vi "PicoScope2000aExampleRapidBlockBulkOverlapped.vi"() -> ()   [LabVIEW 2010]
uses:
  shared/PicoBuffers.ctl
  <vilib>/Waveform/DWDTOps.llb/DWDT Analog to Digital.vi
  shared/Segment Range.ctl
  shared/Buffer and Transfer Settings.ctl
  shared/Acquisition Settings.ctl
  shared/nSegments.ctl
  PicoScope2000aLib/PicoScope2000aDigitalChannelSettings.ctl
  PicoScope2000aLib/PicoScope2000aAnalogChannelSettings.ctl
panel:
  in  "roundFaster":bool=TRUE
  out "Pico 2000a Units":string
  in  "Write to TDMS":bool
  in  "timeIntervalRequested":dbl format="%#6_6p"
  out "Properties Panel":T1 {"Max Total Capture Time Available (sec)" format="%.3p"; "Sample Frequency" format="%.3p"; "Sample Internal" format="%.3p"; "Max Samples Available" format="%.3p"; "Total Capture Time (sec)" format="%.3p"}
  in  "Trigger Settings":T2={"Trigger Enabled"=FALSE, "Trigger Source"=enum."Channel A", "Trigger Threshold (Volts)"=0.0, "Trigger Direction"=2, "Trigger Delay (samples)"=0, "Auto Trigger Time (ms)"=1000} {"Trigger Direction" items=["Rising"=2, "Falling"=3]}
  in  "Channel A Settings":T3={"Enabled"=TRUE, "Coupling"=1, "Range"=6, "Analogue Offset"=0.0} {"Analogue Offset" format="%#_6p"; "Range" items=["20 mV"=1, "50 mV"=2, "100 mV"=3, "200 mV"=4, "500 mV"=5, "1 V"=6, "2 V"=7, "5 V"=8, "10 V"=9, "20 V"=10]; "Coupling" items=["AC", "DC"]}
  out "Device Info":T4={"Driver Version"="0", "USB Version"="0", "Hardware"="0", "Variant"="0", "Batch and Serial"="0", "Cal Date"="0", "Kernel Version"="0", "Digital HW Version"="0", "Analogue HW Version"="0", "Firmware 1"="0", "Firmware 2"="0", "MSO"=FALSE, "Number of Channels"=0}
  out "overflow":i16[](array[numeric]) format="%06b"
  in  "Port 0 Settings":T5={"Enabled"=FALSE, "Logic Level"=9830} {"Logic Level" items=["1.5V TTL"=9830, "2.5V CMOS"=16383]}
  in  "Stop Display":bool
  out "Capture Complete":bool
  in  "Run":bool
  in  "Display Buffer Index":i32
  in  "Segment Range":T6={"fromSegmentIndex"=0, "toSegmentIndex"=9} {"toSegmentIndex" format="%.4p"; "fromSegmentIndex" format="%.4p"}
  in  "nSegments":T7=10 format="%.4p"
  out "error out":errorcluster
  in  "Data file":path=path "PicoScope2000aExampleRapidBlock Data"
  in  "Buffer and Transfer Settings":T8={"startIndex"=0, "Samples"=1000, "Down Sample Ratio"=1, "Down-Sample Mode"=0} {"Down-Sample Mode" items=["RAW none"=2147483648, "None"=0, "Aggregate"=1, "Decimate"=2, "Average"=4]; "Down Sample Ratio" step=1; "Samples" format="%_6p"}
  in  "Acquisition Settings":T9={"preTriggerSamples"=0, "postTriggerSamples"=1000, "timebase"=0} {"postTriggerSamples" format="%_6p"; "preTriggerSamples" format="%_6p"}
  out "Port 0":digitalwaveform(graph)={"t0"=timestamp(0 s since 1904-01-01), "dt"=4.800000041882413e-08, "Y"={"transitions"=[], "data"=[]}}
  in  "stop":bool
  out "Analog Channels":cluster{i32, sgl, "Data":dbl[]}[](graph)
  in  "Serial Number":string
  in  "Use Serial Number":bool
  in  "error in (no error)":errorcluster
  # "Number of\nSegments to Capture"
  # "Bit 0 = ChA"
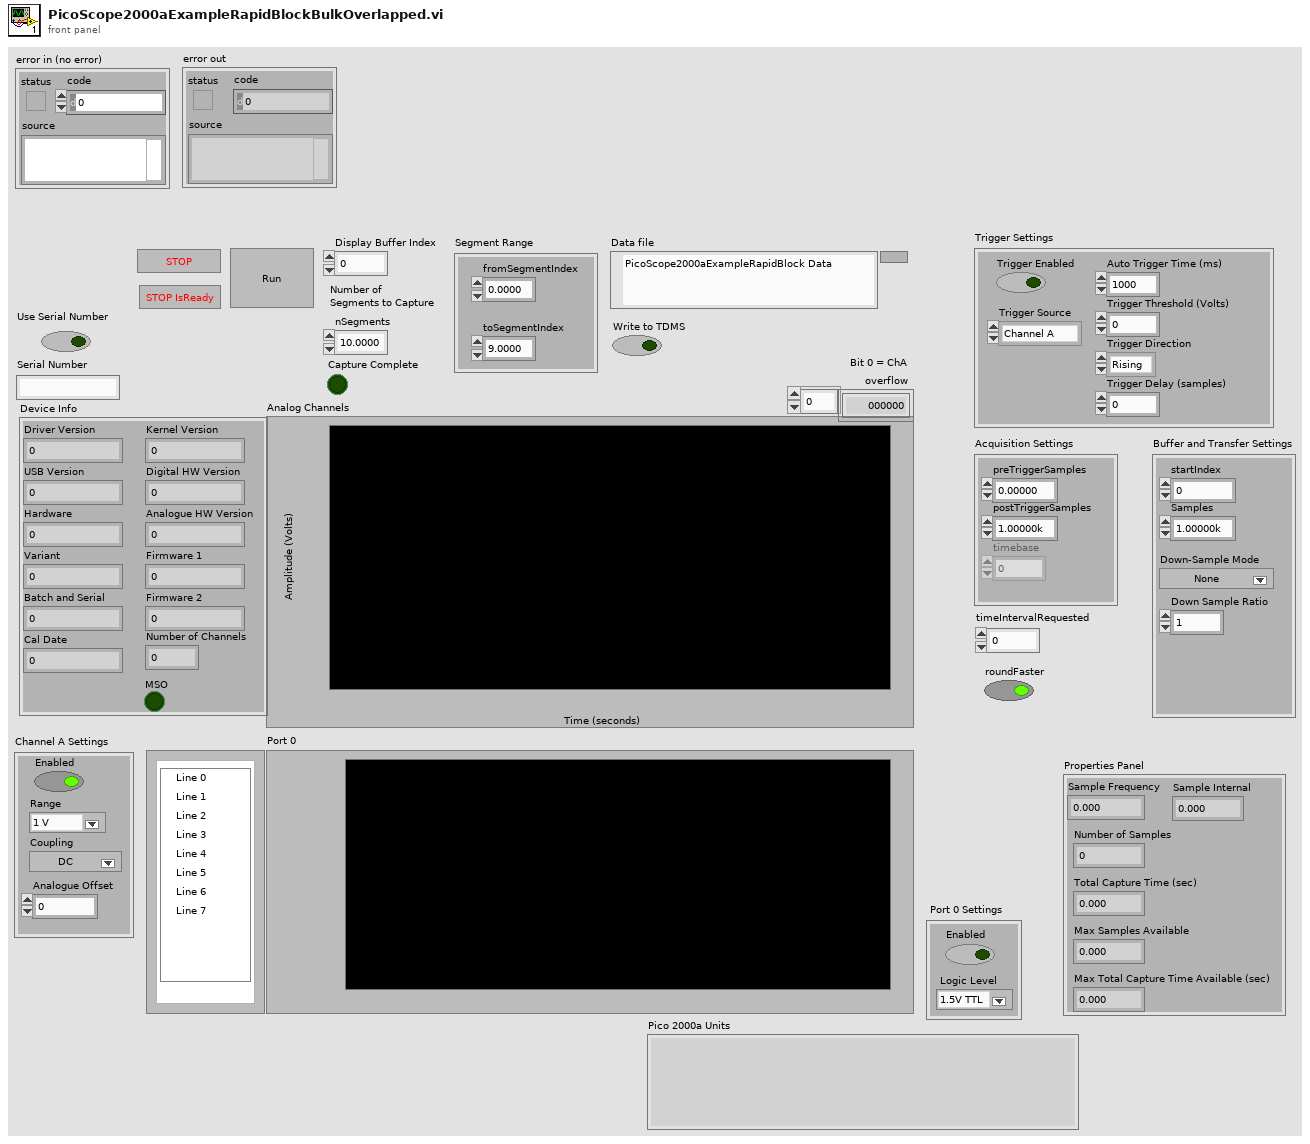
[diagram p1: front panel]
types:
  T1 = cluster{"Sample Frequency":sgl, "Sample Internal":sgl, "Max Samples Available":i32, "Number of Samples":u32, "Total Capture Time (sec) ":sgl, "Max Total Capture Time Available (sec)":sgl}
  T2 = cluster{"Trigger Enabled":bool, "Trigger Source":enum16{"Channel A", "Channel B", "Channel C", "Channel D", "Ext."}, "Trigger Threshold (Volts)":dbl, "Trigger Direction":u16, "Trigger Delay (samples)":u32, "Auto Trigger Time (ms)":i16}
  T3 = typedef "PicoScope2000aAnalogChannelSettings.ctl" = cluster{"Enabled":bool, "Coupling":i16, "Range":u32, "Analogue Offset":sgl}
  T4 = cluster{"Driver Version":string, "USB Version":string, "Hardware":string, "Variant":string, "Batch and Serial":string, "Cal Date":string, "Kernel Version":string, "Digital HW Version":string, "Analogue HW Version":string, "Firmware 1":string, "Firmware 2":string, "MSO":bool, "Number of Channels":i16}
  T5 = typedef "PicoScope2000aDigitalChannelSettings.ctl" = cluster{"Enabled":bool, "Logic Level":i16}
  T6 = typedef "Segment Range.ctl" = cluster{"fromSegmentIndex":u64, "toSegmentIndex":u64}
  T7 = typedef "nSegments.ctl" = u64
  T8 = typedef "Buffer and Transfer Settings.ctl" = cluster{"startIndex":u64, "Samples":u64, "Down Sample Ratio":u64, "Down-Sample Mode":u32}
  T9 = typedef "Acquisition Settings.ctl" = cluster{"preTriggerSamples":u64, "postTriggerSamples":u64, "timebase":u32}
  T10 = typedef "PicoBuffers.ctl" = cluster{"Max Buffer Pointers":u64[][][], "Min Buffer Pointers":u64[][][], "StreamingDataInfo":cluster{"Channel":u32, "Down-Sample Mode":u32, "PICO_DATA_TYPE":enum32{"PICO_INT8_T", "PICO_INT16_T", "PICO_INT32_T", "PICO_UINT32_T", "PICO_INT64_T", ""}, "Samples":i32, "bufferIndex":u64, "startIndex":i32, "overflow":i16}[][]}
  T11 = enum16{"open", "open or create", "create or replace", "create", "open (read-only)"}
  T12 = cluster{"Channel A Buffer":i16[], "Channel B Buffer":i16[], "Channel C Buffer":i16[], "Channel D Buffer":i16[], "Channel E Buffer":i16[], "Channel F Buffer":i16[], "Channel G Buffer":i16[], "Channel H Buffer":i16[], "Port 0 Buffer":i16[], "Port 1 Buffer":i16[]}[]
  T13 = cluster{"Channel A Buffer":i16[], "Channel B Buffer":i16[], "Channel C Buffer":i16[], "Channel D Buffer":i16[], "Channel E Buffer":i16[], "Channel F Buffer":i16[], "Channel G Buffer":i16[], "Channel H Buffer":i16[], "Port 0 Buffer":i16[], "Port 1 Buffer":i16[]}
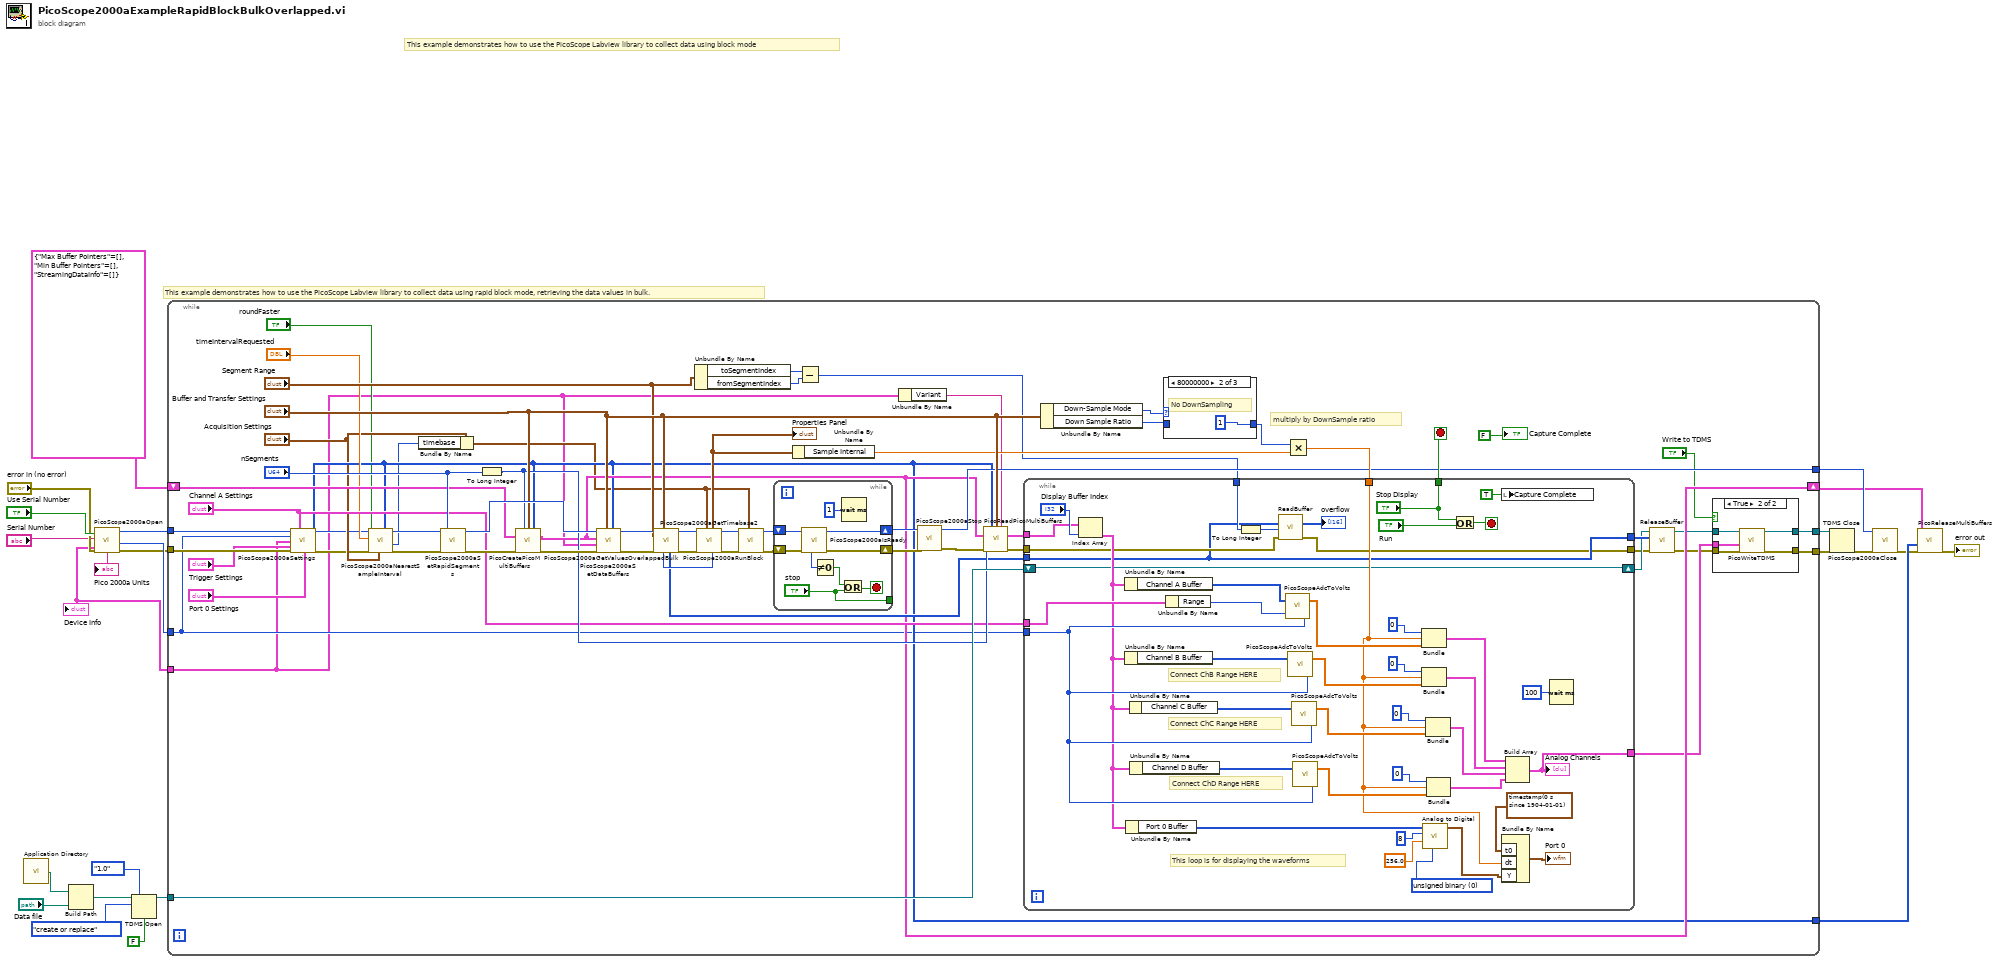
[diagram p0: block diagram]
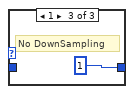
[diagram p4: hidden frame]
diagram:
  # "This example demonstrates how to use the PicoScope Labview library to collect data using rapid block mode, retrieving the data values in bulk."
  # "This example demonstrates how to use the PicoScope Labview library to collect data using block mode"
  n1 = call <vilib>:"Application Directory.vi"() -> ("Application Directory"=w17:path)
  n2 = Build Path(base path=w17, name or relative path="Data file") -> (appended path=w18:path)
  n3 = call "PicoScope2000aOpen.vi"("Serial Number"="Serial Number", "Use Serial Number"="Use Serial Number", "error in (no error)"="error in (no error)") -> ("error out"=w6:errorcluster, "Max Adc value"=w8:i16, "Device Info"=w5:T4, "handle"=w7:i16, "Pico 2000a Units"=→"Pico 2000a Units":string)  [unwired: 3 in, 1 out]
  "Device Info" <- w5
  n4 = TDMS Open(6:FALSE ("disable buffering? (T)"), 7:enum16{"1.0", "2.0"}."1.0" ("file format version (2.0)"), 10:T11."create or replace" ("operation (0:open)"), 11:w18) -> (3:w16:refnum<k34>)  [unwired: 2 in, 1 out]
  n5 = while {
    tunnel: w8 -> [w36]
    tunnel: [w67] -> w23
    tunnel: [w44] -> w24
    tunnel: w16 -> [w86]
    tunnel: [w26] -> w2
    shift-right: [w48] -> w9
    shift-left: T10 {"Max Buffer Pointers"=[], "Min Buffer Pointers"=[], "StreamingDataInfo"=[]} ("Data Pointers") -> [w49]
    tunnel: w7 -> [w38]
    tunnel: w6 -> [w37]
    tunnel: w5 -> [w32]
    tunnel: [w25] -> w3
    stop <- w72 stop-if-true
    # "multiply by DownSample ratio"
    n6 = call "PicoScope2000aSettings.vi"("handle in"=w38, "Channel A Settings"="Channel A Settings", "Max_adc"=w36, "Device Info"=w32, "Trigger Settings"="Trigger Settings", "error in"=w37, "Port 0 Settings"="Port 0 Settings") -> ("handle out"=w39:i16, "Enabled Array"=w44:i16[], "error out"=w40:errorcluster)  [unwired: 6 in]
    n7 = call "PicoScope2000aNearestSampleInterval.vi"("Enabled array"=w44, "Acquisition Settings"="Acquisition Settings", "error in (no error)"=w40, "roundFaster"="roundFaster", "timeIntervalRequested"="timeIntervalRequested", "handle in"=w39) -> ("error out"=w47:errorcluster, "timebase"=w42:u32, "handle out"=w46:i16)  [unwired: 2 in, 1 out]
    n8 = Bundle By Name(cluster="Acquisition Settings", "timebase"=w42) -> (w41:T9)
    n9 = call "PicoScope2000aSetRapidSegments.vi"("nSegments"="nSegments", "error in (no error)"=w47, "handle in"=w46) -> ("error out"=w85:errorcluster, "handle out"=w84:i16)  [unwired: 6 in, 1 out]
    n10 = To Long Integer(number="nSegments") -> (32bit integer=w65:i32)
    n11 = call "PicoCreatePicoMultiBuffers.vi"("Number of Buffers"=w65, "Buffer and Transfer Settings"="Buffer and Transfer Settings", "enabled array"=w44, "Data Pointers In"=w49, "error in (no error)"=w85) -> ("Data Pointers"=w48:T10, "error out"=w87:errorcluster)  [unwired: 9 in]
    n12 = call "PicoScope2000aSetDataBuffers.vi"("enabled array"=w44, "Buffer and Transfer Settings"="Buffer and Transfer Settings", "error in (no error)"=w87, "Device Info"=w32, "Data Pointers In"=w48, "handle in"=w84) -> ("error out"=w83:errorcluster, "handle out"=w82:i16)  [unwired: 4 in]
    n13 = call "PicoScope2000aGetValuesOverlappedBulk.vi"("Segment Range"="Segment Range", "Buffer and Transfer Settings"="Buffer and Transfer Settings", "error in (no error)"=w83, "handle in"=w82) -> ("error out"=w60:errorcluster, "handle out"=w57:i16, "Pointer to Overflow"=w55:u64[], "noOfSamples"=w56:u64)  [unwired: 4 in]
    n14 = Unbundle By Name("Segment Range") -> ("toSegmentIndex"=w53:u64, "fromSegmentIndex"=w52:u64)
    n15 = call "PicoScope2000aGetTimebase2.vi"("Number of Samples"=w56, "Acquisition Settings"=w41, "error in (no error)"=w60, "handle in"=w57) -> ("error out"=w59:errorcluster, "handle out"=w58:i16, "Properties Panel"=w61:T1)  [unwired: 5 in]
    "Properties Panel" <- w61
    n16 = call "PicoScope2000aRunBlock.vi"("Acquisition Settings"=w41, "error in (no error)"=w59, "handle in"=w58) -> ("error out"=w75:errorcluster, "handle out"=w74:i16)  [unwired: 5 in, 2 out]
    n17 = while {
      shift-right: [w145] -> w69
      shift-left: w75 -> [w146]
      shift-right: [w144] -> w66
      shift-left: w74 -> [w143]
      tunnel: ["stop"] -> _
      stop <- w140 stop-if-true
      n18 = call "PicoScope2000aIsReady.vi"("error in (no error)"=w146, "handle in"=w143) -> ("error out"=w145:errorcluster, "handle out"=w144:i16, "ready"=w142:i16)  [unwired: 7 in]
      n19 = Not Equal To 0?(x=w142) -> (x != 0?=w141:bool)
      n20 = Or(x=w141, y="stop") -> (x .or. y?=w140:bool)
      n21 = Wait (ms)(milliseconds to wait=u32 1) -> ()  [unwired: 1 out]
    }
    n22 = Unbundle By Name(w61) -> ("Sample Internal"=w64:sgl)
    n23 = Subtract(x=w53, y=w52) -> (x-y=w50:u64)
    n24 = Unbundle By Name(w32) -> ("Variant"=w63:string)
    n25 = call "PicoScope2000aStop.vi"("error in (no error)"=w69, "handle in"=w66) -> ("error out"=w68:errorcluster, "handle out"=w67:i16)  [unwired: 8 in]
    n26 = call "PicoReadPicoMultiBuffers.vi"("enabled array"=w44, "Buffer and Transfer Settings"="Buffer and Transfer Settings", "Variant"=w63, "Data Pointers"=w48, "No of Buffers"=w65, "error in (no error)"=w68) -> ("MultiBuffers (Max or non-aggregated)"=w80:T12, "error out"=w73:errorcluster)  [unwired: 7 in, 1 out]
    n27 = Unbundle By Name("Buffer and Transfer Settings") -> ("Down-Sample Mode"=w78:u32, "Down Sample Ratio"=w79:u64)
    n28 = case shown="80000000" w78 {
      tunnel: [w147 u64 1 ("Down Sample Ratio") u64 1 ("Down Sample Ratio")] -> w76
      tunnel: w79 -> [w147 _ _]
      frame Default {
      }
      frame -2147483648 {
        # "No DownSampling"
      }
      frame 1 {
        # "No DownSampling"
      }
    }
    n29 = Multiply(x=w76, y=w64) -> (x*y=w77:sgl)
    n30 = while {
      tunnel: w36 -> [w104]
      tunnel: "Channel A Settings" -> [w137]
      tunnel: w80 -> [w114]
      tunnel: w77 -> [w106]
      shift-right: [w95] -> w29
      shift-left: w86 -> [w95]
      tunnel: w73 -> [w100]
      tunnel: ["Stop Display"] -> w72
      tunnel: w55 -> [w98]
      tunnel: [w98] -> w54
      tunnel: w50 -> [w99]
      tunnel: [w97] -> w31
      tunnel: [w96] -> w28
      stop <- w117 stop-if-true
      w128 = u16 0 items=["unsigned binary", "offset binary", "2's complement"] ("data format (offset binary)")
      # "This loop is for displaying the waveforms"
      # "Connect ChB Range HERE"
      # "Connect ChD Range HERE"
      # "Connect ChC Range HERE"
      n31 = Index Array(array=w114, index="Display Buffer Index") -> (element=w103:T13)
      n32 = Unbundle By Name(w103) -> ("Channel A Buffer"=w121:i16[])
      n33 = Unbundle By Name(w103) -> ("Channel B Buffer"=w133:i16[])
      n34 = Unbundle By Name(w103) -> ("Port 0 Buffer"=w126:i16[])
      n35 = Unbundle By Name(w103) -> ("Channel C Buffer"=w112:i16[])
      n36 = Unbundle By Name(w103) -> ("Channel D Buffer"=w108:i16[])
      n37 = Unbundle By Name(w137) -> ("Range"=w135:u32)
      n38 = To Long Integer(number=w99) -> (32bit integer=w102:i32)
      n39 = call "ReadBuffer.vi"("Pointer and BufferSize"=w98, "Buffer size"=w102, "error in (no error)"=w100) -> ("Output Array"=→"overflow":i16[], "error out"=w96:errorcluster)  [unwired: 11 in]
      n40 = call "PicoScopeAdcToVolts.vi"("Max_adc"=w104, "Range Index"=w135, "Data"=w121) -> ("Data"=w122:dbl[])
      n41 = call "PicoScopeAdcToVolts.vi"("Max_adc"=w104, "Data"=w133) -> ("Data"=w132:dbl[])  [unwired: 1 in]
      n42 = call "PicoScopeAdcToVolts.vi"("Max_adc"=w104, "Data"=w112) -> ("Data"=w111:dbl[])  [unwired: 1 in]
      n43 = call "PicoScopeAdcToVolts.vi"("Max_adc"=w104, "Data"=w108) -> ("Data"=w107:dbl[])  [unwired: 1 in]
      n44 = Bundle(0, w106, "Data"=w122) -> (w131:cluster{i32, sgl, "Data":dbl[]})  [unwired: 1 in]
      n45 = Bundle(0, w106, "Data"=w132) -> (w130:cluster{i32, sgl, "Data":dbl[]})  [unwired: 1 in]
      n46 = call-poly <vilib>:"Analog to Digital.vi"("data format (offset binary)"=w128, "full-scale range (pk-pk)"=256.0, "resolution (16 bit)"=8, "analog waveform"=w126) -> ("digital waveform"=w123:digitalwaveform)  [unwired: 4 in, 3 out]
      n47 = Bundle(0, w106, "Data"=w111) -> (w110:cluster{i32, sgl, "Data":dbl[]})  [unwired: 1 in]
      n48 = Bundle(0, w106, "Data"=w107) -> (w105:cluster{i32, sgl, "Data":dbl[]})  [unwired: 1 in]
      n49 = Or(x="Stop Display", y="Run") -> (x .or. y?=w117:bool)
      n50 = local write "Capture Complete"(TRUE ("Capture Complete")) -> ()
      n51 = Bundle By Name("t0"=timestamp(0 s since 1904-01-01), "dt"=w106, "Y"=w123) -> (→"Port 0":digitalwaveform)  [unwired: 1 in]
      n52 = Build Array(w131, w130, w110, w105) -> (w97:cluster{i32, sgl, "Data":dbl[]}[])
      "Analog Channels" <- w97
      n53 = Wait (ms)(milliseconds to wait=u32 100) -> ()  [unwired: 1 out]
    }
    n54 = call "ReleaseBuffer.vi"("error in (no error)"=w28, "Pointer and BufferSize"=w54) -> ("error out"=w27:errorcluster)  [unwired: 9 in]
    n55 = case shown="True" "Write to TDMS" {
      tunnel: w31 -> [_ w94]
      tunnel: w29 -> [w88 w93]
      tunnel: w27 -> [w89 w92]
      tunnel: [w89 w91] -> w26
      tunnel: [w88 w90] -> w25
      frame False {
      }
      frame True {
        n56 = call "PicoWriteTDMS.vi"("error in (no error)"=w92, "Analog Channels"=w94, "Refnum in"=w93) -> ("error out"=w91:errorcluster, "Refnum out"=w90:refnum<k34>)  [unwired: 7 in]
      }
    }
    "Capture Complete" <- FALSE ("Capture Complete")
  }
  n57 = TDMS Close(8:w2, 11:w3) -> (0:w1:errorcluster)  [unwired: 1 out]
  n58 = call "PicoScope2000aClose.vi"("error in (no error)"=w1, "handle in"=w23) -> ("error out"=w11:errorcluster)  [unwired: 8 in, 1 out]
  n59 = call "PicoReleaseMultiBuffers.vi"("error in (no error)"=w11, "Enabled array"=w24, "Data Pointers"=w9) -> ("error out"=→"error out":errorcluster)  [unwired: 7 in, 1 out]
